vi "Fx_Gravity_compensation.vi"(10 "AbsolutePositionRotation":dbl, 11 "Fx_to_filter":dbl) -> (2 "Gravity compensation":dbl(graph), 3 "F_x[N] Gravity compensated":dbl(graph))   [LabVIEW 2019]
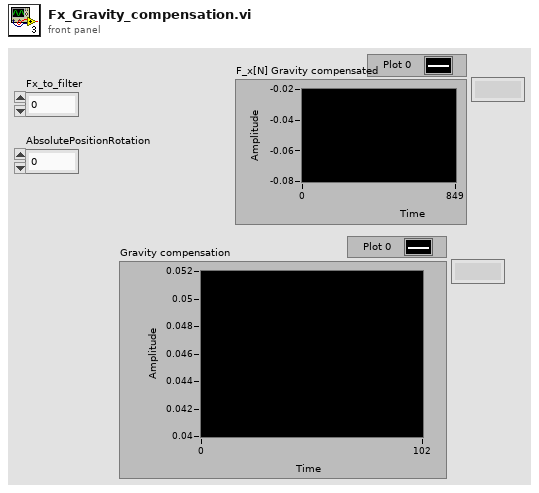
[diagram p1: front panel]
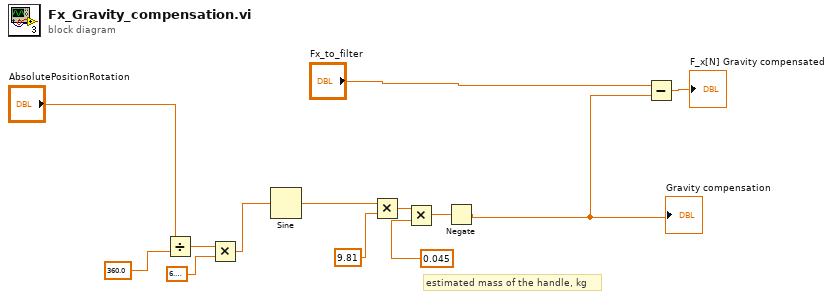
[diagram p0: block diagram]
diagram:
  # "estimated mass of the handle, kg"
  n1 = Divide(x="AbsolutePositionRotation", y=360.0) -> (x/y=w9:dbl)
  n2 = Multiply(x=w9, y=6.283185307179586) -> (x*y=w7:dbl)
  n3 = Sine(x=w7) -> (sin(x)=w6:dbl)
  n4 = Multiply(x=w6, y=9.81) -> (x*y=w5:dbl)
  n5 = Multiply(x=w5, y=0.045 ("mass")) -> (x*y=w2:dbl)
  n6 = Negate(x=w2) -> (-x=w1:dbl)
  "Gravity compensation" <- w1
  n7 = Subtract(x="Fx_to_filter", y=w1) -> (x-y=→"F_x[N] Gravity compensated":dbl)
